vi "Stack.vi"() -> ()   [LabVIEW 2015]
panel:
  out "Iterasi   2":u32
  out "IND":bool
  out "NO 2":u32
  out "OUT 2":u32
  out "NO":u32
  out "Iterasi":u32
  out "OUT":u32
  in  "Stop Button":bool
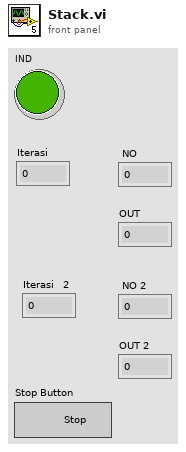
[diagram p1: front panel]
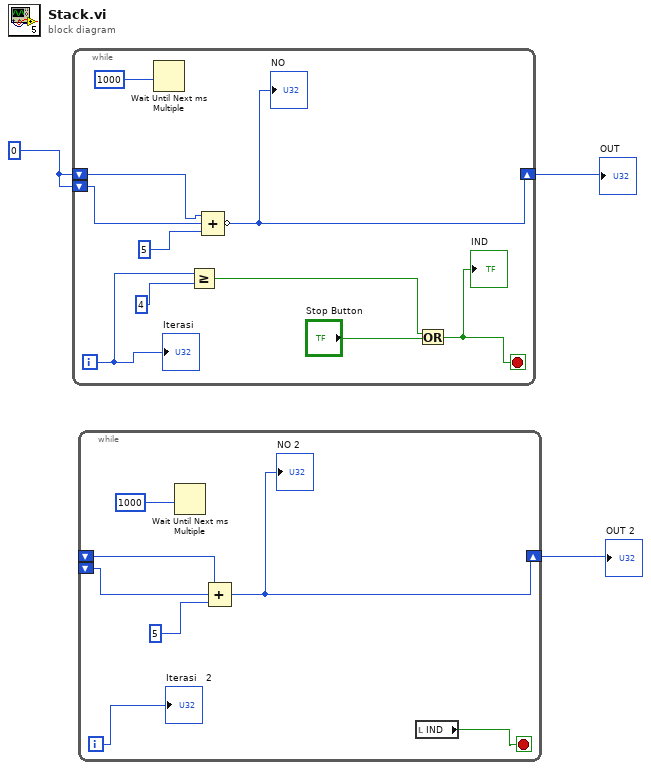
[diagram p0: block diagram]
diagram:
  w3 = 0
  n1 = while {
    shift-right: [w11] -> w2
    shift-left: w3 -> [w7]
    shift-left: w3 -> [w12]
    i -> [w9]
    stop <- w4 stop-if-true
    n2 = Wait Until Next ms Multiple(millisecond multiple=1000) -> ()  [unwired: 1 out]
    n3 = Greater Or Equal?(x=w9, y=4) -> (x >= y?=w5:bool)
    n4 = Compound Arithmetic op=ADD(w7, w12, 5) -> (invert w11:i32)
    "NO" <- w11
    n5 = Or(x=w5, y="Stop Button") -> (x .or. y?=w4:bool)
    "IND" <- w4
    "Iterasi" <- w9
  }
  "OUT" <- w2
  n6 = while {
    shift-right: [w17] -> w1
    shift-left: _ -> [w19]
    shift-left: _ -> [w18]
    i -> [w14]
    stop <- w15 stop-if-true
    n7 = Wait Until Next ms Multiple(millisecond multiple=1000) -> ()  [unwired: 1 out]
    n8 = Compound Arithmetic op=ADD(w19, w18, 5) -> (w17:i32)
    "NO 2" <- w17
    n9 = local read "IND"() -> (w15:bool)
    "Iterasi   2" <- w14
  }
  "OUT 2" <- w1
